vi "ATA_RT_2017_08_07.vi"() -> ()   [LabVIEW 2018]
doc: "This VI transfers a finite number of samples from the FPGA target to the Host using a stream."
uses:
  <vilib>/rvi/interface/nirviMethod/nirviMethod.xnode
  <vilib>/rvi/interface/nirviOpenFPGA/nirviOpenFPGA.xnode
  <vilib>/rvi/interface/nirviCloseFPGA/nirviCloseFPGA.xnode
  <vilib>/rvi/errors/niLvFpgaMergeErrorWithErrorCode.vi
  <vilib>/rvi/interface/nirviReadWriteControl/nirviReadWriteControl.xnode
  <vilib>/FPGAPlugInAG/Dynamic/niLvFpga_ReadFifo_Dynamic.vi
  <vilib>/rvi/Analysis/host/Public/NI_FpgaMspHost.lvlib
  <vilib>/FPGAPlugInAG/Dynamic/niLvFpga_StartFifo_Dynamic.vi
  <vilib>/rvi/interface/Simulation/niFpgaSimulationCallBeginRW.vi
  <vilib>/rvi/errors/niLvFpgaAdjustHostInterfaceError.vi
  <vilib>/Utility/error.llb/Error Cluster From Error Code.vi
  NiFpgaLv.dll
  Controls/DataClass.ctl
  Controls/ToneInfoClust.ctl
  <vilib>/FPGAPlugInAG/Dynamic/niLvFpga_Reset_Dynamic.vi
  <vilib>/FPGAPlugInAG/Dynamic/niLvFpga_Run_Dynamic.vi
  ProjectFiles/FPGA Bitfiles/20171006_01_ATA_FPGA_01.lvbitx
  <vilib>/FPGAPlugInAG/Dynamic/niLvFpga_ConfigureFifo_Dynamic.vi
  <vilib>/FPGAPlugInAG/Dynamic/niLvFpga_Close_Dynamic.vi
  <vilib>/DAQmx/write.llb/DAQmx Write (Digital 1D Bool NChan 1Samp 1Line).vi
  <vilib>/DAQmx/create/channels.llb/DAQmx Create Channel (DO-Digital Output).vi
  <vilib>/FPGAPlugInAG/PXIe-7976R/niLvFpga_Open_PXIe-7976R.vi
  <vilib>/rvi/interface/common/dynamic/niFpgaDynamicAddResources.vi
panel:
  in  "refnum out":refnum<k20>
  in  "?":T1 {"median" format="%0.2f"; "MaxQ" format="%0.2f"}
  out "error out 2":errorcluster
  out "NoiseFloor":dbl format="%^#.1g"
  out "error out":errorcluster
  out "Log Error":errorcluster
  in  "Green":bool
  in  "Blue":bool
  in  "Red":bool
  out "FreqShiftTab":enum32{"Auto", "Manual"}(tab)=enum."Manual"
  in  "CoarseShift":dbl(slide)=-24999000.0 caption="Frequency Shift Coarse (Hz)" scale=-26000000.0..-23000000.0 scale format="%^#_6g"
  in  "FineShift":dbl(slide)=-462.63345195729516 caption="Frequency Shift Fine (Hz)" scale=-10000.0..10000.0 scale format="%^#_6g"
  in  "Beacon_ManualShift":dbl format="%^#_10e"
  in  "ProbesTab":T2(tab)=enum."Settings"
  in  "#Avg":u16=1
  in  "index to remove":i32[](array[numeric])=[0, 1633]
  in  "AvgAvg":bool
  in  "EnableStep1":bool=TRUE
  in  "ScaleMeasurement":fxp<+/-,23,23>=10000.0
  in  "Scale_In_RT":ext=1.0
  in  "Scale_Step1":fxp<+/-,23,23>=4194303.0
  in  "Scale_NoiseFloor":fxp<+/-,23,23>=4194303.0
  in  "Offset":fxp<+/-,16,1>=0.000213623046875
  in  "FlushQ":bool=TRUE
  in  "Enable":T3={"FreqShiftEnable"=TRUE, "Step4Enable"=TRUE, "Step5Enable"=TRUE, "Step6Enable"=TRUE, "Step7Enable"=TRUE}
  in  "Scale":T4={"Scale_Step4"=10.0, "Scale_Step5"=1.0, "Scale_Step6"=1.0, "Scale_Step7"=1.0}
  out "NoiseFloorFIFOTimeOut":bool
  out "ReceiverTimed Out":bool
  out "#Transfers":i32=74
  out "#FFTs":i32=74
  out "Elements Remaining":u32
  out "Peak Location Cal":dbl=25000106.633451957 format="%^#_11g"
  out "SampleRate":dbl=12500.0
  out "max value Beacon":dbl=4.648353358875404e-06
  out "max index Beacon":i32=644
  out "FAM Initialized?":bool=TRUE
  out "CalShift":dbl=-24999462.633451957
  out "BeaconShift":dbl
  out "# elements in DSP queue":i32
  out "Peak Location Beacon":dbl
  out "MaxIndexCal":i32
  out "MaxValue Cal":dbl
  in  "AutoCenter":bool
  in  "Tab Control 2":T5(tab)
  out "TimeDomainBeacon":ext[](graph)
  out "TimeDomainCal":ext[](graph)
  out "df (Hz)":dbl=1.0
  in  "Zoom On Peak":bool
  in  "Tones":u8(slide)=1 scale=0.0..1.0
  out "Filtered Spectrum Cal":dbl[](graph)
  out "Filtered Spectrum Beacon":dbl[](graph)
  out "NoiseFloor":dbl[](graph)
  out "df (Hz) 2":dbl=7629.39453125
  out "NoiseFloorLoopCount":i32=77
  in  "Noise Floor":u8(slide)=1 scale=0.0..1.0
  in  "stop":bool
  # "Log"
  # "Linear"
  # "Log"
  # "Linear"
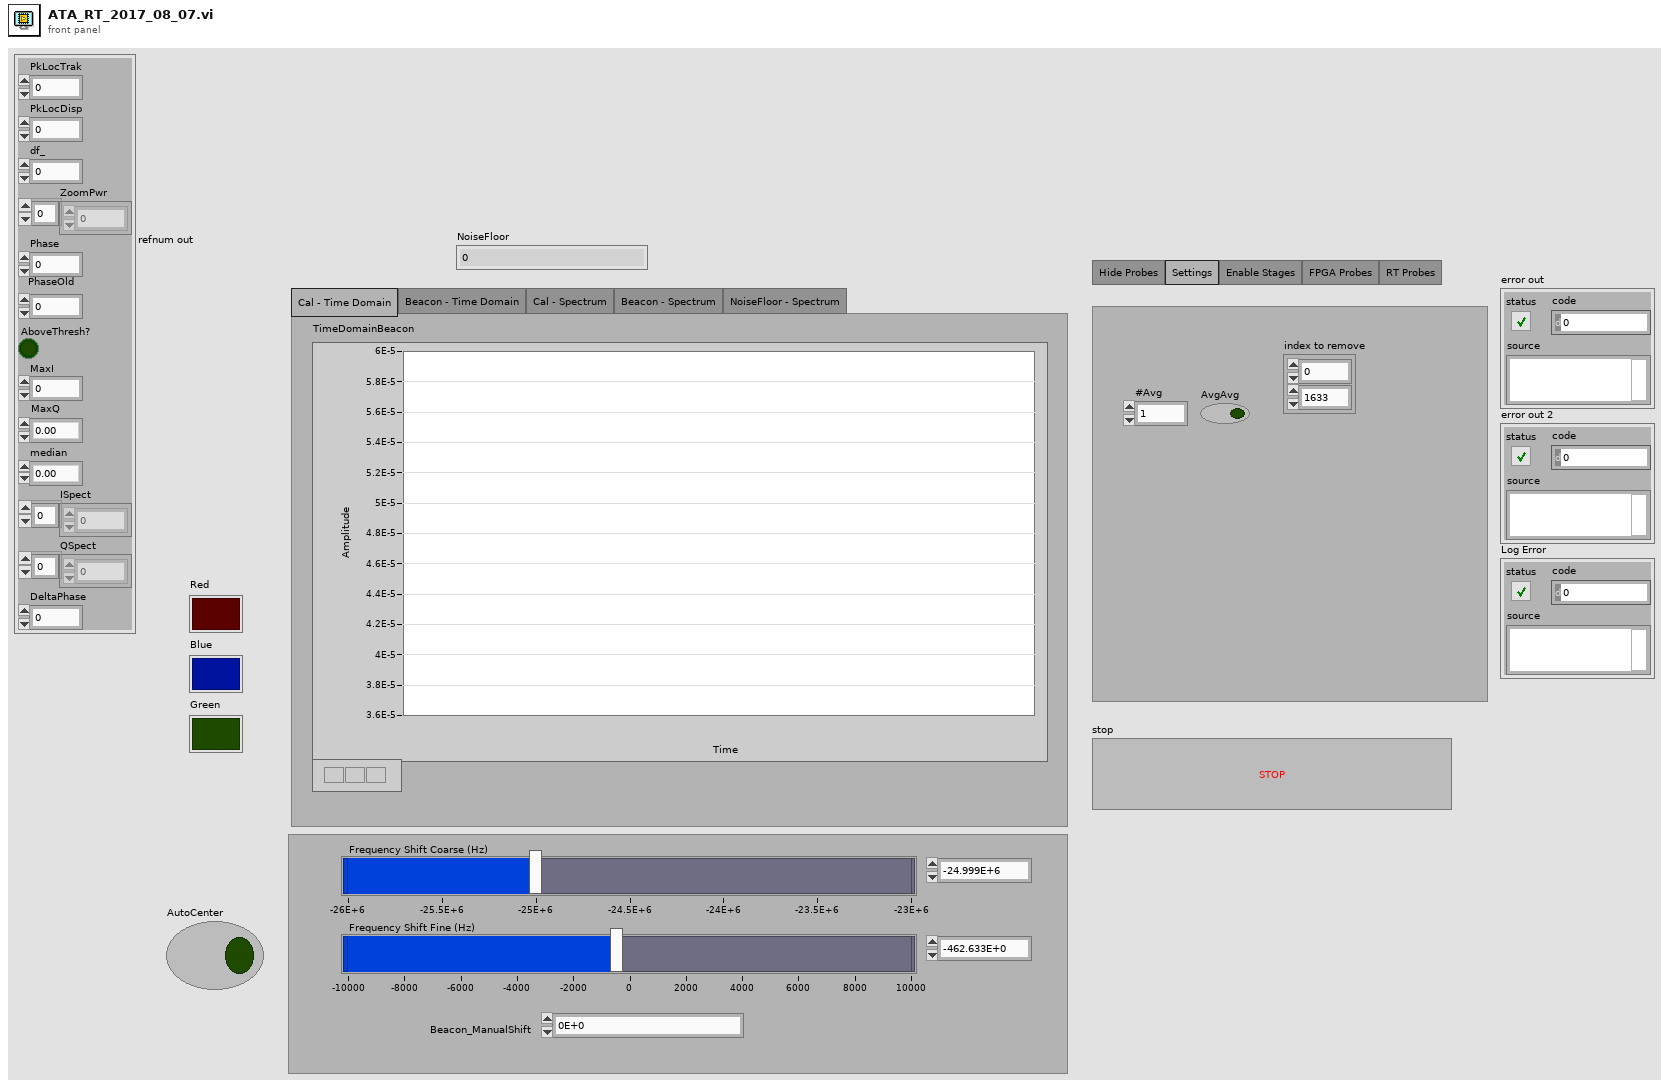
[diagram p1: front panel]
types:
  T1 = typedef "ToneInfoClust.ctl" = cluster{"PkLocTrak":dbl, "PkLocDisp":dbl, "df_":dbl, "ZoomPwr":dbl[], "Phase":dbl, "PhaseOld":dbl, "AboveThresh?":bool, "MaxI":dbl, "MaxQ":dbl, "median":dbl, "ISpect":dbl[], "QSpect":dbl[], "DeltaPhase":dbl}
  T2 = enum32{"Hide Probes", "Settings", "Enable Stages", "FPGA Probes", "RT Probes"}
  T3 = cluster{"FreqShiftEnable":bool, "Step4Enable":bool, "Step5Enable":bool, "Step6Enable":bool, "Step7Enable":bool}
  T4 = cluster{"Scale_Step4":fxp<+/-,23,23>, "Scale_Step5":fxp<+/-,23,23>, "Scale_Step6":fxp<+/-,23,23>, "Scale_Step7":fxp<+/-,23,23>}
  T5 = enum32{"Cal - Time Domain", "Beacon - Time Domain", "Cal - Spectrum", "Beacon - Spectrum", "NoiseFloor - Spectrum"}
  T6 = enum16{"open", "replace", "create", "open or create", "replace or create", "replace or create with confirmation"}
  T7 = typedef "DataClass.ctl" = enum16{"Tone", "Noise"}
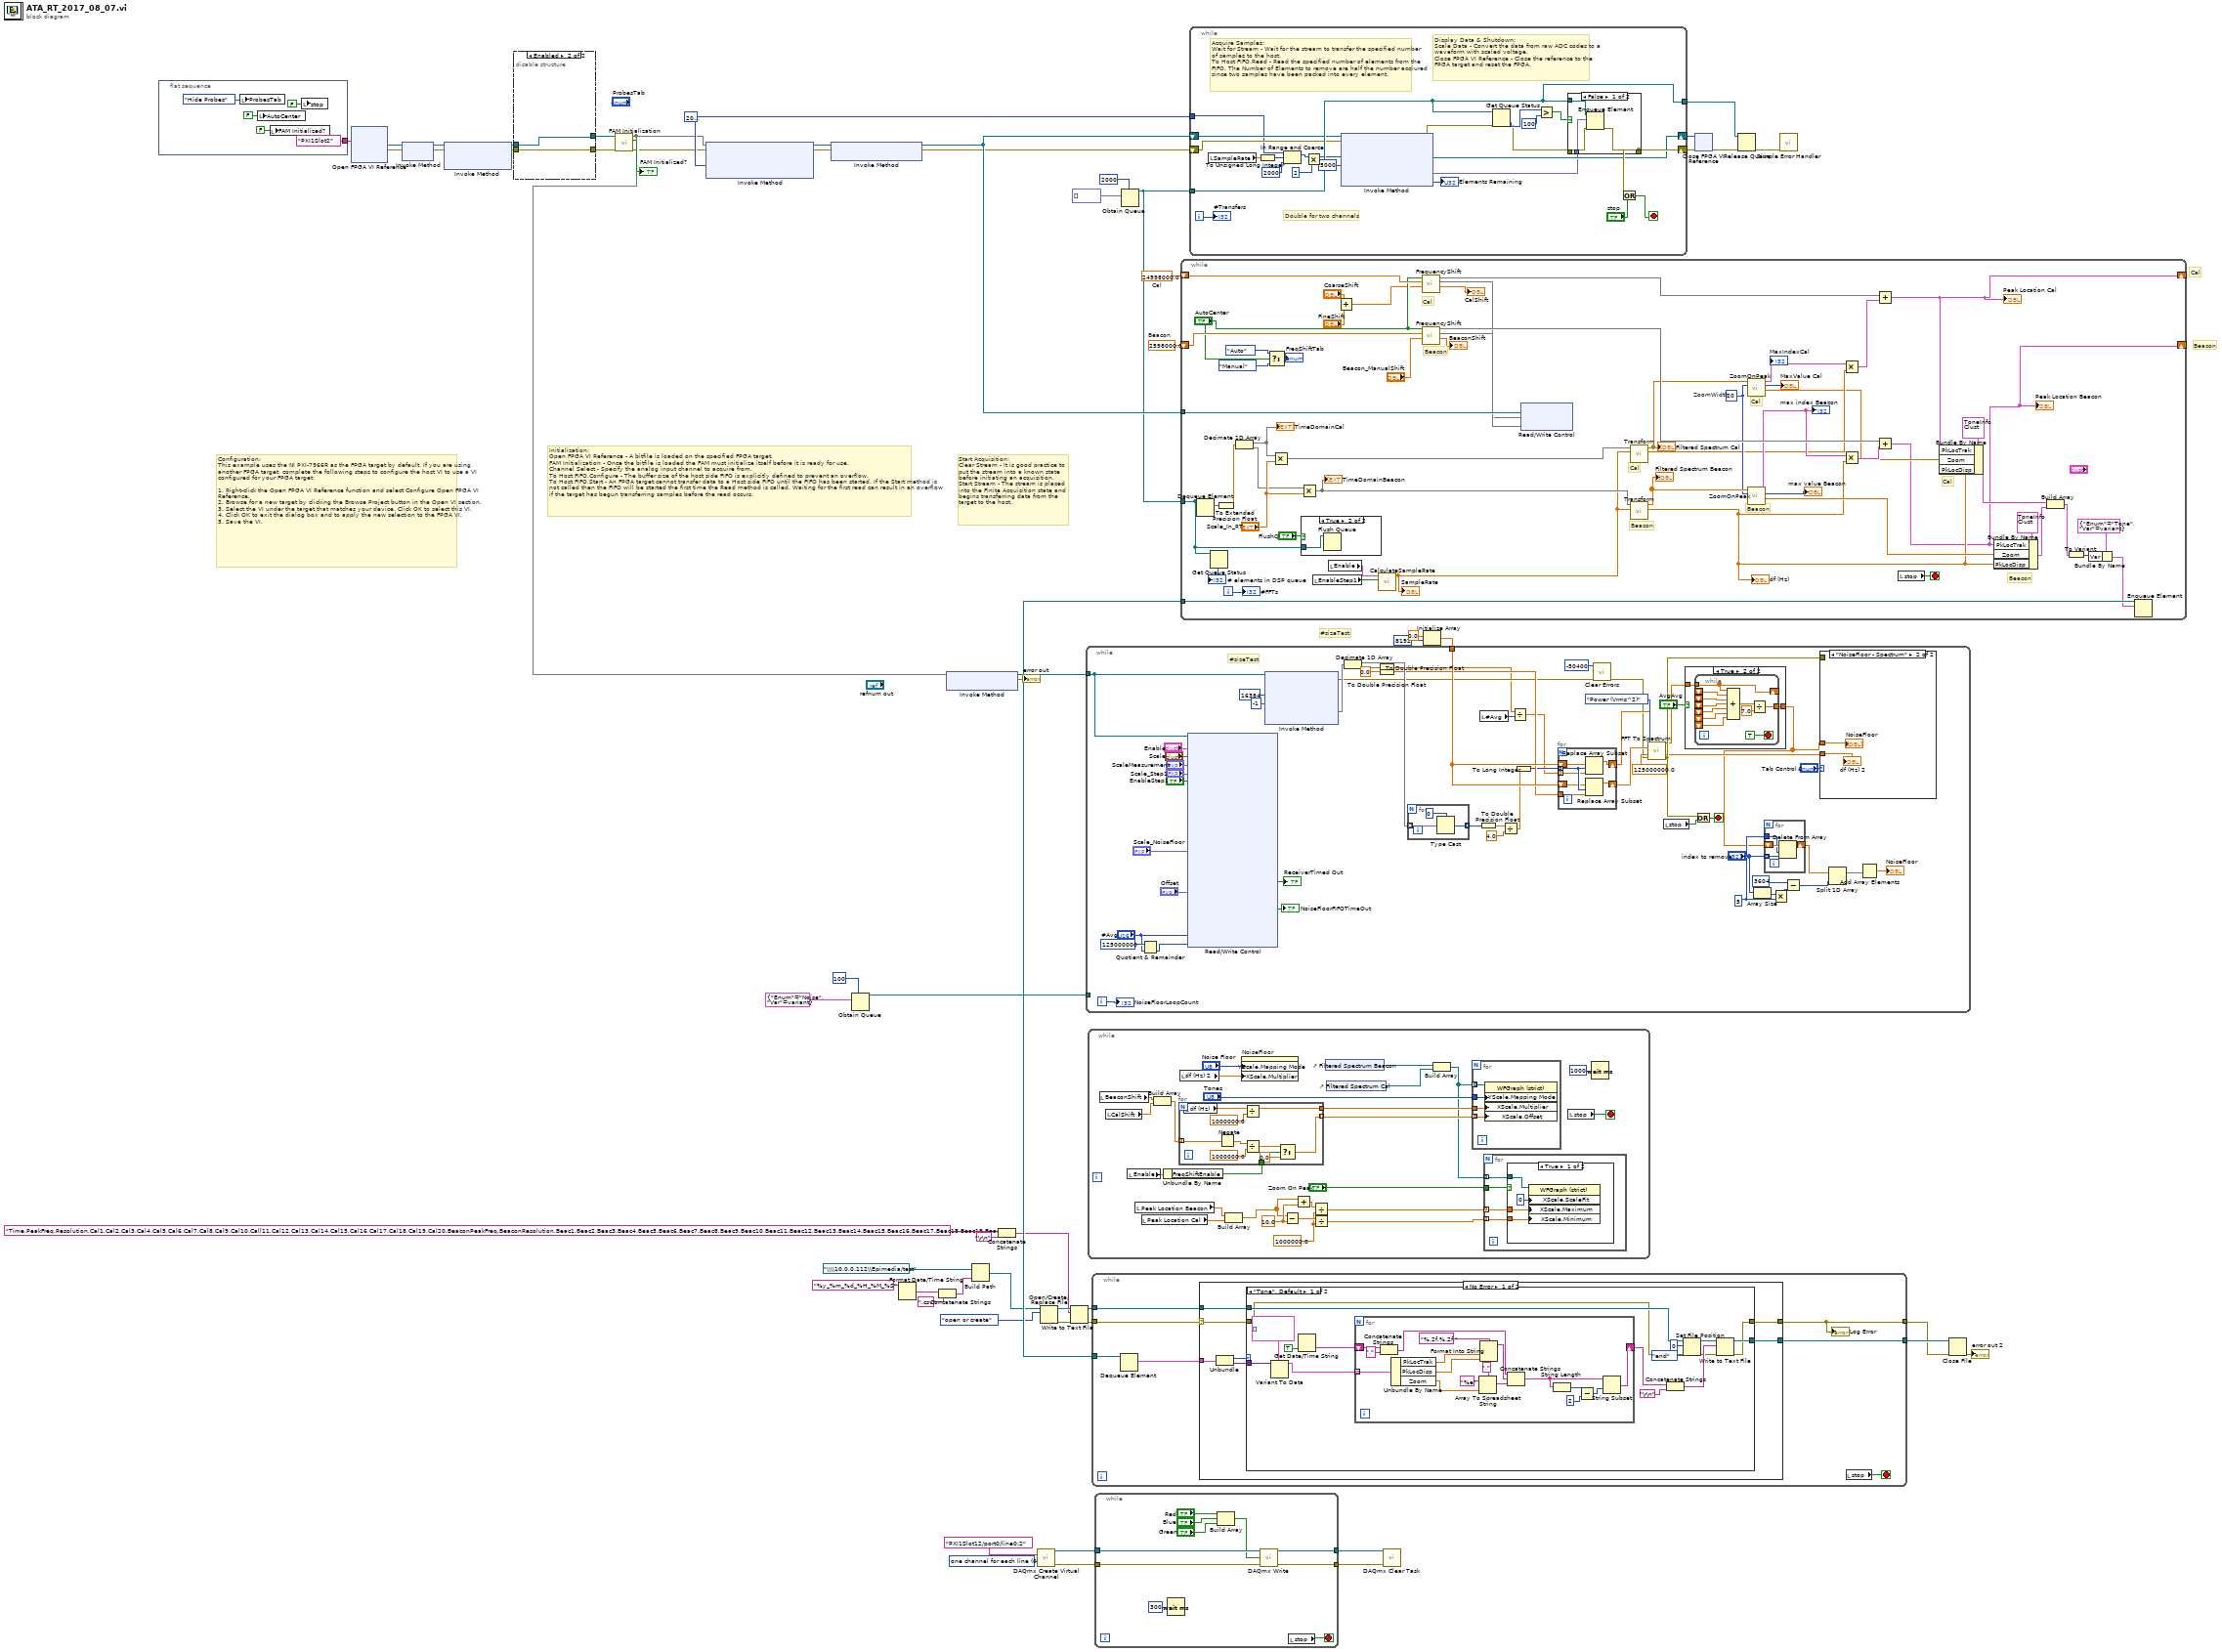
[diagram p0: block diagram]
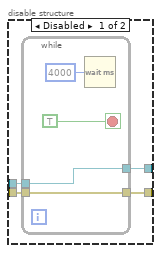
[diagram p2: hidden frame]
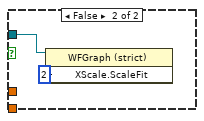
[diagram p5: hidden frame]
diagram:
  w18 = 0 items=["one channel for each line", "one channel for all lines"] ("line grouping")
  w24 = 2598000.0  # Beacon
  w52 = u32 2000000 ("Num Samples")
  w25 = 24998000.0  # Cal
  # "#sizeTest"
  # "Beacon"
  # "Cal"
  # "Start Acquisition:\nClear Stream - It is good practice to put the stream into a known state before initiating an acquisition.\nStart Stream - The stream is placed into the Finite Acquisition state and begins transferring data from the target to the host."
  # "Initialization:\nOpen FPGA VI Reference - A bitfile is loaded on the specified FPGA target.\nFAM Initialization - Once the bitfile is loaded the FAM must initialize itself before it is ready for use.\nChannel Select - Specify the analog input channel to acquire from.\nTo Host FIFO.Configure - The buffer size of the host side FIFO is explicitly defined to prevent an overflow.\nTo Host FIFO.Start - An FPGA target cannot transfer data to a Host side FIFO until the FIFO has been started. If the Start method is not called then the FIFO will be started the first time the Read method is called. Waiting for the first read can result in an overflow if the target has begun transferring samples before the read occurs."
  # "Configuration:\nThis example uses the NI PXI-7966R as the FPGA target by default. If you are using another FPGA target, complete the following steps to configure the host VI to use a VI configured for your FPGA target:\n\n1. Right-click the Open FPGA VI Reference function and select Configure Open FPGA VI Reference.\n2. Browse for a new target by clicking the Browse Project button in the Open VI section.\n3. Select the VI under the target that matches your device. Click OK to select this VI.\n4. Click OK to exit the dialog box and to apply the new selection to the FPGA VI.\n5. Save the VI."
  n1 = flat-sequence {
    tunnel: [tag "PXI1Slot2" ("resource name")] -> w45
    frame #0 {
      n2 = local write "ProbesTab"(T2."Hide Probes" ("ProbesTab")) -> ()
      n3 = local write "AutoCenter"(FALSE ("AutoCenter")) -> ()
      n4 = local write "FAM Initialized?"(FALSE ("FAM Initialized?")) -> ()
      n5 = local write "stop"(FALSE ("stop")) -> ()
    }
  }
  n6 = xnode ("Open FPGA VI Reference")("resource name"=w45) -> ("FPGA VI Reference Out"=w11:refnum<k20>, "error out"=w10:errorcluster)  [unwired: 1 in]
  n7 = xnode "Invoke Method"("FPGA VI Reference In"=w11, "error in"=w10) -> ("FPGA VI Reference Out"=w2:refnum<k20>, "error out"=w1:errorcluster)
  n8 = xnode "Invoke Method"("FPGA VI Reference In"=w2, "error in"=w1) -> ("FPGA VI Reference Out"=w6:refnum<k20>, "error out"=w5:errorcluster)  [unwired: 1 in]
  n9 = disable-structure shown="Enabled" {
    disable-tunnel: [w67 w72] -> w9
    disable-tunnel: [w66 w73] -> w8
    disable-tunnel: w6 -> [w65 w73]
    disable-tunnel: w5 -> [w64 w72]
    frame Disabled {
      n10 = while {
        tunnel: [w69] -> w67
        tunnel: w64 -> [w69]
        tunnel: [w68] -> w66
        tunnel: w65 -> [w68]
        stop <- TRUE ("Start") stop-if-true
        n11 = Wait (ms)(milliseconds to wait=u32 4000) -> ()  [unwired: 1 out]
      }
    }
    frame Enabled {
    }
  }
  n12 = call "FAM Initialization.vi"("error in (no error)"=w9, "Cluster"=w8) -> ("error out"=w38:errorcluster, "FAM Initialized?"=→"FAM Initialized?":bool, 3:w39)  [unwired: 7 in]
  n13 = xnode "Invoke Method"("FPGA VI Reference In"=w39, "error in"=w38, "Requested Depth"=w52) -> ("FPGA VI Reference Out"=w57:refnum<k20>, "error out"=w56:errorcluster)  [unwired: 1 out]
  n14 = xnode "Invoke Method"("FPGA VI Reference In"=w57, "error in"=w56) -> ("FPGA VI Reference Out"=w55:refnum<k20>, "error out"=w37:errorcluster)
  n15 = Obtain Queue(max queue size (-1, unlimited)=100, element data type=cluster{"Enum":T7, "Var":variant} {"Enum"=enum."Noise", "Var"=variant}) -> (queue out=w42:refnum<queue>)  [unwired: 3 in, 2 out]
  n16 = Format Date/Time String(time format string (%c)="%y_%m_%d_%H_%M_%S") -> (date/time string=w31:string)  [unwired: 2 in]
  n17 = Concatenate Strings(w31, ".csv" ("string")) -> (w33:string)
  n18 = xnode "Invoke Method"("FPGA VI Reference In"=w39) -> ("FPGA VI Reference Out"=w12:refnum<k20>, "error out"=→"error out":errorcluster)  [unwired: 1 in]
  n19 = Build Path(base path=path "\\\\10.0.0.112\\Epimedia/test" ("file (use dialog)"), name or relative path=w33) -> (appended path=w35:path)
  n20 = Concatenate Strings("Time,PeakFreq,Resolution,Cal1,Cal2,Cal3,Cal4,Cal5,Cal6,Cal7,Cal8,Cal9,Cal10,Call11,Cal12,Cal13,Cal14,Cal15,Cal16,Cal17,Cal18,Cal19,Cal20,BeaconPeakFreq,BeaconResolution,Beac1,Beac2,Beac3,Beac4,Beac5,Beac6,Beac7,Beac8,Beac9,Beac10,Beac11,Beac12,Beac13,Beac14,Beac15,Beac16,Beac17,Beac18,Beac19,Beac20" ("text"), "\r\n") -> (w27:string)
  n21 = call-poly <vilib>:"DAQmx Create Virtual Channel.vi"("lines"=tag "PXI1Slot12/port0/line0:2", "line grouping"=w18) -> ("task out"=w22:refnum<k21>, "error out"=w21:errorcluster)  [unwired: 12 in]
  n22 = Open/Create/Replace File(file path (use dialog)=w35, operation (0:open)=T6."open or create") -> (refnum out=w30:refnum<file>, error out=w17:errorcluster)  [unwired: 4 in, 1 out]
  n23 = Write to Text File(file (use dialog)=w30, text=w27, error in=w17) -> (refnum out=w29:refnum<file>, error out=w16:errorcluster)  [unwired: 1 in, 1 out]
  n24 = while {
    stop <- w98 stop-if-true
    w86 = 1000000.0 ("x")
    w92 = 10.0 ("y")
    n25 = local read "BeaconShift"() -> (w79:dbl)
    n26 = local read "CalShift"() -> (w78:dbl)
    n27 = local read "Enable"() -> (w84:T3)
    n28 = local read "Peak Location Beacon"() -> (w74:dbl)
    n29 = local read "Peak Location Cal"() -> (w75:dbl)
    n30 = Build Array(w79, w78) -> (w77:dbl[])
    n31 = Unbundle By Name(w84) -> ("FreqShiftEnable"=w83:bool)
    n32 = for {
      tunnel: [w107] -> w93
      tunnel: [w102] -> w85 mode=indexing
      tunnel: w83 -> [w101]
      tunnel: w77 -> [w99] mode=indexing
      n33 = local read "df (Hz)"() -> (w108:dbl)
      n34 = Negate(x=w99) -> (-x=w105:dbl)
      n35 = Divide(x=w108, y=1000000.0) -> (x/y=w107:dbl)
      n36 = Divide(x=w105, y=1000000.0) -> (x/y=w103:dbl)
      n37 = Select(t=w103, s=w101, f=0.0) -> (s? t:f=w102:dbl)
    }
    n38 = local read "df (Hz) 2"() -> (w94:dbl)
    n39 = Build Array(w74, w75) -> (w76:dbl[])
    n40 = property on="NoiseFloor" class="WFGraph (strict)"("YScale.Mapping Mode"="Noise Floor", "XScale.Multiplier"=w94) -> ()  [unwired: 2 in, 2 out]
    n41 = Subtract(x=w76, y=w92) -> (x-y=w88:dbl[])
    n42 = Add(x=w76, y=w92) -> (x+y=w91:dbl[])
    n43 = Divide(x=w91, y=w86) -> (x/y=w89:dbl[])
    n44 = Divide(x=w88, y=w86) -> (x/y=w87:dbl[])
    n45 = control-ref of="Filtered Spectrum Beacon"() -> (w82:refnum<vi>)
    n46 = control-ref of="Filtered Spectrum Cal"() -> (w81:refnum<vi>)
    n47 = Build Array(w82, w81) -> (w80:refnum<vi>[])
    n48 = for {
      tunnel: "Tones" -> [w122]
      tunnel: w93 -> [w121]
      tunnel: w85 -> [w120] mode=indexing
      tunnel: w80 -> [w119] mode=indexing
      n49 = property on="Property Node" class="WFGraph (strict)"(reference=w119, "YScale.Mapping Mode"=w122, "XScale.Multiplier"=w121, "XScale.Offset"=w120) -> ()  [unwired: 1 in, 2 out]
    }
    n50 = for {
      tunnel: "Zoom On Peak" -> [w112]
      tunnel: w89 -> [w111] mode=indexing
      tunnel: w87 -> [w110] mode=indexing
      tunnel: w80 -> [w109] mode=indexing
      n51 = case shown="True" w112 {
        tunnel: w110 -> [w116 _]
        tunnel: w111 -> [w115 _]
        tunnel: w109 -> [w113 w117]
        frame True {
          n52 = property on="Property Node" class="WFGraph (strict)"(reference=w113, "XScale.ScaleFit"=u8 0 ("X Scale.Scale Fit"), "XScale.Maximum"=w115, "XScale.Minimum"=w116) -> ()  [unwired: 1 in, 2 out]
        }
        frame False {
          n53 = property on="Property Node" class="WFGraph (strict)"(reference=w117, "XScale.ScaleFit"=u8 2 ("X Scale.Scale Fit")) -> ()  [unwired: 1 in, 2 out]
        }
      }
    }
    n54 = local read "stop"() -> (w98:bool)
    n55 = Wait (ms)(milliseconds to wait=u32 1000) -> ()  [unwired: 1 out]
  }
  n56 = while {
    tunnel: w42 -> [w125]
    tunnel: w29 -> [w127]
    tunnel: [w126] -> w41
    tunnel: w16 -> [w124]
    tunnel: [w123] -> w4
    stop <- w129 stop-if-true
    n57 = Dequeue Element(queue=w125) -> (element=w128:cluster{"Enum":T7, "Var":variant})  [unwired: 2 in, 3 out]
    n58 = case shown="No Error" w124 {
      selector: w124 -> [w131 w172]
      tunnel: w128 -> [w136 _]
      tunnel: w127 -> [w133 w173]
      tunnel: [w132 w173] -> w126
      tunnel: [w130 w172] -> w123
      frame No Error {
        n59 = Unbundle(w136) -> ("Enum"=w135:T7, "Var"=w134:variant)
        n60 = case shown="\"Tone\", Default" w135 {
          tunnel: w134 -> [w152 _]
          tunnel: w133 -> [w150 w171]
          tunnel: [w146 w171] -> w132
          tunnel: w131 -> [w139 w170]
          tunnel: [w137 w170] -> w130
          frame "Tone", Default {
            n61 = Variant To Data(type=T1[] [] ("appended array"), Variant=w152) -> (data=w151:T1[])  [unwired: 1 in, 1 out]
            n62 = Get Date/Time String(want seconds? (F)=TRUE) -> (time string=w140:string)  [unwired: 2 in, 1 out]
            n63 = for {
              tunnel: w151 -> [w169] mode=indexing
              shift-right: [w159] -> w144
              shift-left: w140 -> [w154]
              n64 = Concatenate Strings(w154, "," ("string")) -> (w153:string)
              n65 = Unbundle By Name(w169) -> ("PkLocTrak"=w164:dbl, "PkLocDisp"=w162:dbl, "Zoom"=w165:dbl[])
              n66 = Array To Spreadsheet String(delimiter (Tab)=",", array=w165, 3:"%e" ("format string")) -> (spreadsheet string=w166:string)
              n67 = Format Into String(format string="%.2f,%.2f,", w164, w162) -> (resulting string=w163:string)  [unwired: 2 in, 1 out]
              n68 = Concatenate Strings(w153, w163, w166) -> (w160:string)
              n69 = String Length(string=w160) -> (length=w158:i32)
              n70 = Subtract(x=w158, y=2 ("x")) -> (x-y=w157:i32)
              n71 = String Subset(string=w160, length (rest)=w157) -> (substring=w159:string)  [unwired: 1 in]
            }
            n72 = Concatenate Strings(w144, "\r\n") -> (w143:string)
            n73 = Set File Position(offset (in bytes) (0)=i64 0, refnum=w150, from (0:start)=enum16{"start", "end", "current"}."end", error in=w139) -> (refnum out=w149:refnum<file>, error out=w138:errorcluster)
            n74 = Write to Text File(file (use dialog)=w149, text=w143, error in=w138) -> (refnum out=w146:refnum<file>, error out=w137:errorcluster)  [unwired: 1 in, 1 out]
          }
          frame "Noise" {
          }
        }
      }
      frame Error {
      }
    }
    "Log Error" <- w123
    n75 = local read "stop"() -> (w129:bool)
  }
  n76 = while {
    tunnel: w22 -> [w183]
    tunnel: w21 -> [w182]
    tunnel: [w180] -> w19
    tunnel: [w179] -> w20
    stop <- w181 stop-if-true
    n77 = Wait (ms)(milliseconds to wait=u32 300) -> ()  [unwired: 1 out]
    n78 = Build Array("Red", "Blue", "Green") -> (w174:bool[])
    n79 = call-poly <vilib>:"DAQmx Write.vi"("task/channels in"=w183, "data"=w174, "error in"=w182) -> ("task out"=w179:refnum<k21>, "error out"=w180:errorcluster)  [unwired: 10 in, 1 out]
    n80 = local read "stop"() -> (w181:bool)
  }
  n81 = Obtain Queue(max queue size (-1, unlimited)=2000, element data type=fxp<+/-,40,1>[] [] ("Data")) -> (queue out=w49:refnum<queue>)  [unwired: 3 in, 2 out]
  n82 = while {
    tunnel: w49 -> [w184]
    tunnel: w55 -> [w237]
    shift-right: [w186] -> _
    shift-left: w24 -> [w227]
    tunnel: w42 -> [w219]
    shift-right: [w187] -> _
    shift-left: w25 -> [w212]
    i -> [w226]
    stop <- w239 stop-if-true
    w206 = 20  # ZoomWidth
    # "Cal"
    # "Beacon"
    # "Beacon"
    # "Cal"
    # "Beacon"
    # "Cal"
    # "Cal"
    # "Beacon"
    n83 = Dequeue Element(queue=w184) -> (element=w236:fxp<+/-,40,1>[])  [unwired: 2 in, 3 out]
    n84 = Get Queue Status(queue=w184) -> (# elements in queue=→"# elements in DSP queue":i32)  [unwired: 2 in, 7 out]
    n85 = To Extended Precision Float(1:w236) -> (0:w213:ext[])
    n86 = Decimate 1D Array(w213) -> (w205:ext[], w204:ext[])
    "TimeDomainCal" <- w205
    n87 = Select(t=enum32{"Auto", "Manual"}."Auto" ("FreqShiftTab"), s="AutoCenter", f=enum32{"Auto", "Manual"}."Manual" ("FreqShiftTab")) -> (s? t:f=→"FreqShiftTab":enum32{"Auto", "Manual"})
    n88 = Multiply(x=w205, y="Scale_In_RT") -> (x*y=w208:ext[])
    n89 = Multiply(x=w204, y="Scale_In_RT") -> (x*y=w235:ext[])
    "TimeDomainBeacon" <- w235
    n90 = case shown="True" "FlushQ" {
      tunnel: w184 -> [_ w240]
      frame False {
      }
      frame True {
        n91 = Flush Queue(queue=w240) -> ()  [unwired: 1 in, 3 out]
      }
    }
    n92 = local read "EnableStep1"() -> (w232:bool)
    n93 = local read "Enable"() -> (w222:T3)
    n94 = Add(x="CoarseShift", y="FineShift") -> (x+y=w190:dbl)
    n95 = call "CalculateSampleRate.vi"("Radio Buttons"=w232, 11:w222) -> ("f"=w210:dbl)  [unwired: 9 in]
    "SampleRate" <- w210
    n96 = call "FrequencyShift.vi"("Shift_"=w190, "NewestPeak"=w212, "Tone.AboveThresh?"="AutoCenter") -> ("TotalShift"=→"CalShift":dbl, 2:w192, 3:w199)  [unwired: 6 in]
    n97 = call "FrequencyShift.vi"("Shift_"="Beacon_ManualShift", "NewestPeak"=w227, "Tone.AboveThresh?"="AutoCenter") -> ("TotalShift"=→"BeaconShift":dbl, 2:w231, 3:w228)  [unwired: 6 in]
    n98 = xnode "Read/Write Control"("FPGA VI Reference In"=w237, "FreqShiftCal"=w192, "FreqShiftBeac"=w231) -> ()  [unwired: 1 in, 2 out]
    n99 = call "Transform.vi"("SampleRate"=w210, "TimeDomainIn"=w208) -> ("df (Hz)"=w202:dbl, "AmplitudeSpectrum"=w207:dbl[])  [unwired: 4 in, 4 out]
    "Filtered Spectrum Cal" <- w207
    n100 = call "Transform.vi"("SampleRate"=w210, "TimeDomainIn"=w235) -> ("df (Hz)"=w196:dbl, "AmplitudeSpectrum"=w221:dbl[])  [unwired: 4 in, 4 out]
    "df (Hz)" <- w196
    "Filtered Spectrum Beacon" <- w221
    n101 = call "ZoomOnPeak.vi"("ZoomWidth"=w206, "Power spectrum in"=w207) -> ("Power of Peak"=w197:dbl, "MaxIndex"=→"MaxValue Cal":i32, "ZoomQ"=w201:cluster{"ZoomQPos":dbl[], "ZoomQNeg":dbl[]})  [unwired: 4 in, 3 out]
    "MaxIndexCal" <- w201
    n102 = call "ZoomOnPeak.vi"("ZoomWidth"=w206, "Power spectrum in"=w221) -> ("Power of Peak"=w217:dbl, "MaxIndex"=→"max value Beacon":i32, "ZoomQ"=w220:cluster{"ZoomQPos":dbl[], "ZoomQNeg":dbl[]})  [unwired: 4 in, 3 out]
    "max index Beacon" <- w220
    n103 = Multiply(x=w201, y=w202) -> (x*y=w198:cluster{"ZoomQPos":dbl[], "ZoomQNeg":dbl[]})
    n104 = Multiply(x=w220, y=w196) -> (x*y=w229:cluster{"ZoomQPos":dbl[], "ZoomQNeg":dbl[]})
    n105 = Add(x=w199, y=w198) -> (x+y=w187:cluster{"ZoomQPos":dbl[], "ZoomQNeg":dbl[]})
    "Peak Location Cal" <- w187
    n106 = Add(x=w228, y=w229) -> (x+y=w186:cluster{"ZoomQPos":dbl[], "ZoomQNeg":dbl[]})
    "Peak Location Beacon" <- w186
    n107 = local read "stop"() -> (w239:bool)
    n108 = Bundle By Name(cluster=T1 {"PkLocTrak"=0.0, "PkLocDisp"=0.0, "df_"=0.0, "ZoomPwr"=[], "Phase"=0.0, "PhaseOld"=0.0, "AboveThresh?"=FALSE, "MaxI"=0.0, "MaxQ"=0.0, "median"=0.0, "ISpect"=[], "QSpect"=[], "DeltaPhase"=0.0}, "PkLocTrak"=w187, "Zoom"=w197, "PkLocDisp"=w196) -> (w195:T1)
    n109 = Bundle By Name(cluster=T1 {"PkLocTrak"=0.0, "PkLocDisp"=0.0, "df_"=0.0, "ZoomPwr"=[], "Phase"=0.0, "PhaseOld"=0.0, "AboveThresh?"=FALSE, "MaxI"=0.0, "MaxQ"=0.0, "median"=0.0, "ISpect"=[], "QSpect"=[], "DeltaPhase"=0.0}, "PkLocTrak"=w186, "Zoom"=w217, "PkLocDisp"=w196) -> (w194:T1)
    n110 = Build Array(w195, w194) -> (w193:T1[])
    n111 = To Variant(anything=w193) -> (Variant=w215:variant)
    n112 = Bundle By Name(cluster=cluster{"Enum":T7, "Var":variant} {"Enum"=enum."Tone", "Var"=variant} ("element"), "Var"=w215) -> (w214:cluster{"Enum":T7, "Var":variant})
    n113 = Enqueue Element(queue=w219, element=w214) -> ()  [unwired: 2 in, 3 out]
    "#FFTs" <- w226
  }
  n114 = while {
    tunnel: w52 -> [w247]
    shift-right: [w251] -> w54
    shift-left: w55 -> [w252]
    shift-right: [w255] -> w53
    shift-left: w37 -> [w249]
    tunnel: w49 -> [w253]
    tunnel: [w253] -> w47
    i -> [w261]
    stop <- w262 stop-if-true
    # "Double for two channels"
    # "Display Data & Shutdown:\nScale Data - Convert the data from raw ADC codes to a waveform with scaled voltage.\nClose FPGA VI Reference - Close the reference to the FPGA target and reset the FPGA."
    # "Acquire Samples:\nWait for Stream - Wait for the stream to transfer the specified number of samples to the host.\nTo Host FIFO.Read - Read the specified number of elements from the FIFO. The Number of Elements to remove are half the number acqiured since two samples have been packed into every element."
    n115 = local read "SampleRate"() -> (w246:dbl)
    n116 = To Unsigned Long Integer(number=w246) -> (unsigned 32bit integer=w243:u32)
    n117 = In Range and Coerce(upper limit=w247, x=w243, lower limit=u32 2000) -> (coerced(x)=w245:u32)  [unwired: 1 out]
    n118 = Multiply(x=w245, y=u32 2) -> (x*y=w242:u32)
    n119 = xnode "Invoke Method"("FPGA VI Reference In"=w252, "error in"=w249, "Number of Elements"=w242, "Timeout (ms)"=5000) -> ("FPGA VI Reference Out"=w251:refnum<k20>, "error out"=w257:errorcluster, "Data"=w248:fxp<+/-,40,1>[], "Elements Remaining"=→"Elements Remaining":u32)
    n120 = Get Queue Status(queue=w253, error in (no error)=w257) -> (error out=w256:errorcluster, # elements in queue=w259:i32)  [unwired: 1 in, 6 out]
    n121 = Greater?(x=w259, y=100) -> (0:w254:bool)
    n122 = case shown="False" w254 {
      tunnel: w248 -> [w267 _]
      tunnel: w253 -> [w266 _]
      tunnel: w256 -> [w265 w268]
      tunnel: [w264 w268] -> w255
      frame False {
        n123 = Enqueue Element(queue=w266, element=w267, error in (no error)=w265) -> (error out=w264:errorcluster)  [unwired: 1 in, 2 out]
      }
      frame True {
      }
    }
    n124 = Or(x=w255, y="stop") -> (x .or. y?=w262:bool)
    "#Transfers" <- w261
  }
  n125 = call <vilib>:"DAQmx Clear Task.vi"("task in"=w20, "error in"=w19) -> ()  [unwired: 13 in, 1 out]
  n126 = Initialize Array(0.0 ("element"), 8192 ("dimension size")) -> (w13:dbl[])
  n127 = while {
    tunnel: w12 -> [w303]
    tunnel: w42 -> [_]
    tunnel: w13 -> [w298]
    i -> [w320]
    stop <- w318 stop-if-true
    w276 = 5 ("#toRemove")
    # "#sizeTest"
    n128 = Quotient & Remainder(x=u32 125000000, y="#Avg") -> (floor(x/y)=w284:u32)  [unwired: 1 out]
    n129 = xnode "Read/Write Control"("FPGA VI Reference In"=w303, "Enable"="Enable", "Scale"="Scale", "ScaleMeasurement"="ScaleMeasurement", "Scale_Step1"="Scale_Step1", "EnableStep1"="EnableStep1", "Scale_NoiseFloor"="Scale_NoiseFloor", "Offset"="Offset", "#Avg"="#Avg", "SampleCountReset"=w284) -> ("ReceiverTimed Out"=→"ReceiverTimed Out":bool, "NoiseFloorFIFOTimeOut"=→"NoiseFloorFIFOTimeOut":bool)  [unwired: 1 in, 15 out]
    n130 = xnode "Invoke Method"("FPGA VI Reference In"=w303, "Number of Elements"=u32 16384, "Timeout (ms)"=-1) -> ("error out"=w290:errorcluster, "Data"=w309:fxp<+/-,30,15>[])  [unwired: 1 in, 2 out]
    n131 = Decimate 1D Array(w309) -> (w299:fxp<+/-,30,15>[], w308:fxp<+/-,30,15>[])
    n132 = To Double Precision Float(number=w308) -> (double precision float=w283:dbl[])
    n133 = To Double Precision Float(number=0.0) -> (double precision float=w297:dbl)
    n134 = for {
      tunnel: w299 -> [w349] mode=indexing
      tunnel: [w348] -> w292 mode=indexing
      n135 = Type Cast(type=0, x=w349) -> (*(type *) &x=w348:i32)
    }
    n136 = local read "#Avg"() -> (w281:u16)
    n137 = To Double Precision Float(number=w292) -> (double precision float=w302:dbl[])
    n138 = Divide(x=w302, y=4.0) -> (x/y=w294:dbl[])
    n139 = Divide(x=w283, y=w281) -> (x/y=w282:dbl[])
    n140 = To Long Integer(number=w294) -> (32bit integer=w293:i32[])
    n141 = for {
      tunnel: w293 -> [w347] mode=indexing
      shift-right: [w345] -> w295
      shift-left: w298 -> [w346]
      shift-right: [w343] -> w296
      shift-left: w298 -> [w344]
      tunnel: w282 -> [w342] mode=indexing
      tunnel: w297 -> [w341]
      n142 = Replace Array Subset(array=w346, new element=w342, index=w347) -> (w345:dbl[])
      n143 = Replace Array Subset(array=w344, new element=w341, index=w347) -> (w343:dbl[])
    }
    n144 = call <vilib>:"Clear Errors.vi"("error in (no error)"=w290, "specific error code to clear (0: all)"=-50400) -> ("error out"=w289:errorcluster)  [unwired: 4 in, 1 out]
    n145 = call <vilib>:"FFT To Spectrum.vi"("real FFT data"=w295, "imaginary FFT data"=w296, "spectrum type"=enum8{"Power (Vrms^2)", "Amplitude (Vrms)"}."Power (Vrms^2)", "sample rate (S/s)"=125000000.0, "error in (no error)"=w289) -> ("spectrum out"=w271:dbl[], "df (Hz)"=w305:dbl, "error out"=w306:errorcluster)  [unwired: 8 in]
    n146 = local read "stop"() -> (w319:bool)
    n147 = case shown="True" "AvgAvg" {
      tunnel: w271 -> [w323 w325]
      tunnel: [w323 w324] -> w270
      frame False {
      }
      frame True {
        n148 = while {
          shift-right: [w326] -> _
          shift-left: _ -> [w336]
          shift-left: _ -> [w335]
          shift-left: _ -> [w332]
          shift-left: _ -> [w331]
          shift-left: _ -> [w330]
          shift-left: _ -> [w329]
          tunnel: [w328] -> w324
          tunnel: w325 -> [w326]
          stop <- TRUE stop-if-true
          n149 = Compound Arithmetic op=ADD(w326, w336, w335, w332, w331, w330, w329) -> (w334:dbl[])
          n150 = Divide(x=w334, y=7.0) -> (x/y=w328:dbl[])
        }
      }
    }
    n151 = Or(x=w306, y=w319) -> (x .or. y?=w318:bool)
    n152 = Array Size(array="index to remove") -> (size(s)=w277:i32)
    n153 = for {
      tunnel: w276 -> [w338]
      tunnel: "index to remove" -> [w337] mode=indexing
      shift-right: [w339] -> w280
      shift-left: w270 -> [w340]
      n154 = Delete From Array(array=w340, length=w338, index=w337) -> (array with subset deleted=w339:dbl[])  [unwired: 1 out]
    }
    n155 = Multiply(x=w277, y=w276) -> (x*y=w275:i32)
    n156 = Subtract(x=3604 ("index"), y=w275) -> (x-y=w274:i32)
    n157 = case shown="\"NoiseFloor - Spectrum\"" "Tab Control 2" {
      tunnel: w270 -> [_ w352]
      tunnel: w305 -> [_ w351]
      tunnel: w306 -> [_ _]
      frame Default {
      }
      frame "NoiseFloor - Spectrum" {
        "NoiseFloor" <- w352
        "df (Hz) 2" <- w351
      }
    }
    n158 = Split 1D Array(array=w280, index=w274) -> (first subarray=w273:dbl[])  [unwired: 1 out]
    n159 = Add Array Elements(numeric array=w273) -> (sum=→"NoiseFloor":dbl)
    "NoiseFloorLoopCount" <- w320
  }
  n160 = xnode ("Close FPGA VI Reference")("FPGA VI Reference In"=w54, "error in"=w53) -> ("error out"=w51:errorcluster)
  n161 = Release Queue(queue=w47, error in (no error)=w51) -> (error out=w50:errorcluster)  [unwired: 1 in, 2 out]
  n162 = call <vilib>:"Simple Error Handler.vi"("error in (no error)"=w50) -> ()  [unwired: 4 in, 5 out]
  n163 = Close File(refnum=w41, error in=w4) -> (error out=→"error out 2":errorcluster)  [unwired: 1 out]
